vi "Teleop.vi"(10 "Match Info":T1={"Autonomous Elapsed Seconds"=0.0, "TeleOp Elapsed Seconds"=0.0, "Disabled Elapsed Seconds"=0.0, "Visited Autonomous"=FALSE, "Visited TeleOp"=FALSE, "Visited Disabled"=FALSE, "Autonomous Settings"={"Autonomous Style"=enum."Independent", "VI Refnum"=refnum}}, 11 "Call Context":T2) -> ()   [LabVIEW 2016]
doc: "This VI is called for each TeleOp packet received from the DS where the robot is not disabled. It is often used to read from the joysticks and update I/O or to update setpoints for timed control loops. It should complete and return within 20 milliseconds or it may miss DS packets."
uses:
  <vilib>/Rock Robotics/WPI/DriverStation/WPI_DriverStationDerivedRobotMode.ctl
  <vilib>/Rock Robotics/WPI/DriverStation/WPI_DriverStationMatch Info.ctl
  <vilib>/Rock Robotics/WPI/Utilities/WPI_GetSetVariantRefNum.vi
  <vilib>/Rock Robotics/Network Tables/NT Write Numeric Array.vi
  <vilib>/Rock Robotics/Network Tables/NT Read Boolean.vi
  <vilib>/Rock Robotics/Network Tables/NT Write Number.vi
  <vilib>/Rock Robotics/Network Tables/NT Write Boolean.vi
  <vilib>/Rock Robotics/Network Tables/NT Read Number.vi
  <vilib>/Rock Robotics/Network Tables/NT Write Boolean Array.vi
panel:
  out "Limit?":bool
  out "Lift Bottom":dbl
  out "Lift Top":dbl
  out "Sample Boolean 1":bool
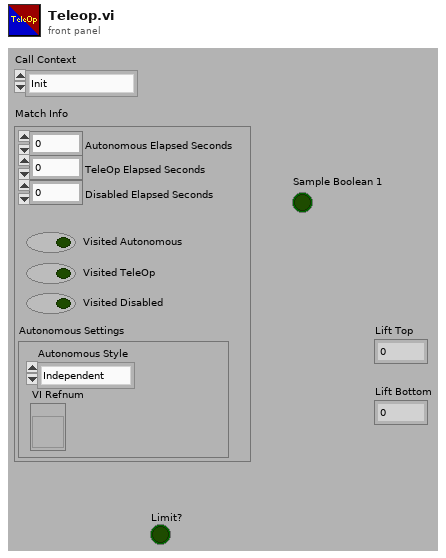
[diagram p1: front panel]
types:
  T1 = typedef "WPI_DriverStationMatch Info.ctl" = cluster{"Autonomous Elapsed Seconds":dbl, "TeleOp Elapsed Seconds":dbl, "Disabled Elapsed Seconds":dbl, "Visited Autonomous":bool, "Visited TeleOp":bool, "Visited Disabled":bool, "Autonomous Settings":cluster{"Autonomous Style":enum16{"Iterative", "Independent"}, "VI Refnum":refnum<vi>}}
  T2 = typedef "WPI_DriverStationDerivedRobotMode.ctl" = enum16{"Init", "Execute", "Stop"}
  T3 = typedef "WPI_GyroDevRef.ctl" = cluster{"DevStatus":errorcluster, "Analog Channel":T4, "Offset":dbl, "Gain (VoltsPerDegree/Second)":dbl, "Gyro Type":enum16{"Analog", "XRS450"}, "Handle":i32, "SPI Bus":T5, "Device Found":bool, "Sample Rate":dbl, "Calibrate On Open":bool}
  T4 = typedef "FPGA_AIChannel.ctl" = enum8{"AI 0", "AI 1", "AI 2", "AI 3", "AI MXP 0", "AI MXP 1", "AI MXP 2", "AI MXP 3", "Invalid"}
  T5 = typedef "spi_bus.ctl" = enum16{"SPI On-Board, CS0", "SPI On-Board, CS1", "SPI On-Board, CS2", "SPI On-Board, CS3", "SPI MXP", "Invalid"}
  T6 = typedef "WPI_JoystickDevRef.ctl" = cluster{"Device":T7}
  T7 = typedef "WPI_JoystickDeviceEnum.ctl" = enum16{"USB 0", "USB 1", "USB 2", "USB 3", "USB 4", "USB 5"}
  T8 = cluster{"Buttons[0]":bool, "Buttons[1]":bool, "Buttons[2]":bool, "Buttons[3]":bool, "Buttons[4]":bool, "Buttons[5]":bool, "Buttons[6]":bool, "Buttons[7]":bool, "Buttons[8]":bool}
  T9 = typedef "WPI_DigitalInputDevRef.ctl" = cluster{"DevStatus":errorcluster, "DIO Channel":T10}
  T10 = typedef "FPGA_DIOChannel.ctl" = enum8{"DIO 0", "DIO 1", "DIO 2", "DIO 3", "DIO 4", "DIO 5", "DIO 6", "DIO 7", "DIO 8", "DIO 9", "DIO MXP 0", "DIO MXP 1", "DIO MXP 2", "DIO MXP 3", "DIO MXP 4", "DIO MXP 5", "DIO MXP 6", "DIO MXP 7", "DIO MXP 8", "DIO MXP 9", "DIO MXP 10", "DIO MXP 11", "DIO MXP 12", "DIO MXP 13", "DIO MXP 14", "DIO MXP 15", "SPI Port CS1", "SPI Port CS2", "SPI Port CS3", "SPI Port MISO", "SPI Port MOSI", "Invalid"}
  T11 = typedef "WPI_RobotDriveDevRef.ctl" = cluster{"DevStatus":errorcluster, "Motors[]":T12[], "Square Inputs":bool, "Max Output":dbl}
  T12 = typedef "WPI_MotorControlDeviceRef.ctl" = cluster{"DeviceStatus":errorcluster, "Type":T13, "PWM":cluster{"PWM Channel":T14, "DeadBand":T15}, "CAN":cluster{"Device Number":u8, "SetOutput VI Ref":variant, "GetOutput VI Ref":variant, "Enable VI Ref":variant, "Disable VI Ref":variant, "Data":variant}, "Invert":bool}
  T13 = typedef "WPI_MotorControlType.ctl" = enum16{"PWM", "CAN"}
  T14 = typedef "FPGA_DIOPWMChannel.ctl" = enum8{"PWM 0", "PWM 1", "PWM 2", "PWM 3", "PWM 4", "PWM 5", "PWM 6", "PWM 7", "PWM 8", "PWM 9", "PWM MXP 0", "PWM MXP 1", "PWM MXP 2", "PWM MXP 3", "PWM MXP 4", "PWM MXP 5", "PWM MXP 6", "PWM MXP 7", "PWM MXP 8", "PWM MXP 9", "Invalid"}
  T15 = typedef "WPI_PWMDeadband.ctl" = cluster{"Name":string, "maxPositivePwm":i32, "minPositivePwm":i32, "centerPwm":i32, "maxNegativePwm":i32, "minNegativePwm":i32, "angularRange":u16}
  T16 = cluster{"Axes[0]":dbl, "Axes[1]":dbl, "Axes[2]":dbl, "Axes[3]":dbl, "Axes[4]":dbl, "Axes[5]":dbl, "Axes[6]":dbl, "Axes[7]":dbl, "Axes[8]":dbl}
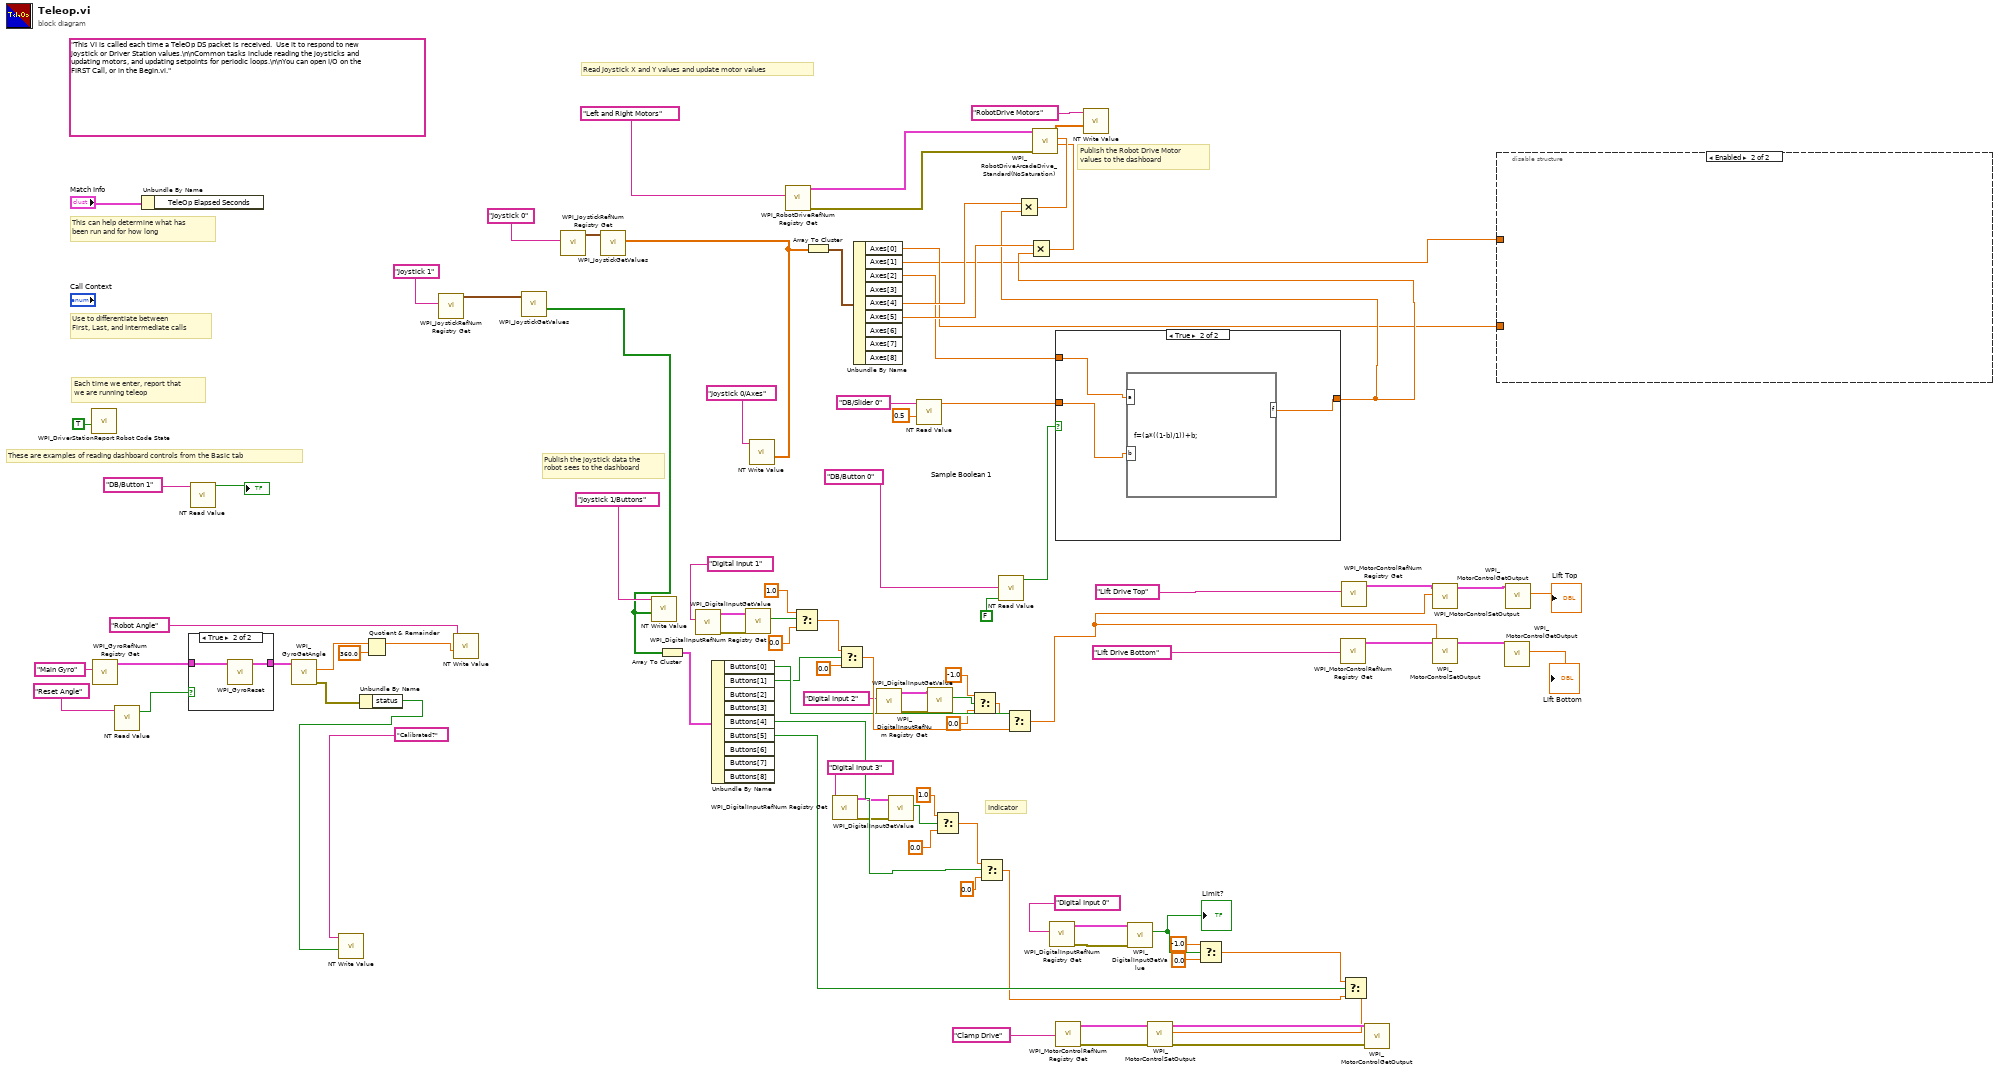
[diagram p0: block diagram]
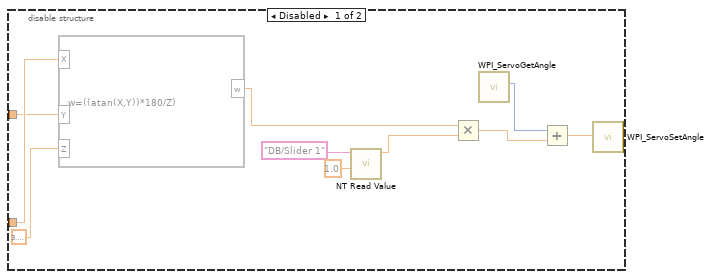
[diagram p2: hidden frame]
diagram:
  (unwired) "This VI is called each time a TeleOp DS packet is received.  Use it to respond to new joystick or Driver Station values.\n\nCommon tasks include reading the joysticks and updating motors, and updating setpoints for periodic loops.\n\nYou can open I/O on the FIRST Call, or in the Begin.vi."
  # "Indicator"
  # "These are examples of reading dashboard controls from the Basic tab"
  # "Publish the Robot Drive Motor\nvalues to the dashboard"
  # "Publish the joystick data the\nrobot sees to the dashboard"
  # "Each time we enter, report that\nwe are running teleop"
  # "Use to differentiate between\nFirst, Last, and Intermediate calls"
  # "This can help determine what has\nbeen run and for how long"
  # "Read Joystick X and Y values and update motor values"
  n1 = call <vilib>:"WPI_DriverStationReport Robot Code State.vi"("TeleOp"=TRUE ("Autonomous")) -> ()  [unwired: 10 in, 1 out]
  n2 = call <vilib>:"WPI_GyroRefNum Registry Get.vi"("refnum name"="Main Gyro") -> ("GyroDevRef"=w61:T3)  [unwired: 9 in, 1 out]
  n3 = call-poly <vilib>:"NT Read Value.vi"("Name"="Reset Angle") -> ("Boolean"=w58:bool)  [unwired: 9 in, 1 out]
  n4 = Unbundle By Name("Match Info") -> ()  [unwired: 1 out]
  n5 = case shown="True" w58 {
    tunnel: [w97 w99] -> w65
    tunnel: w61 -> [w97 w98]
    frame False {
    }
    frame True {
      n6 = call <vilib>:"WPI_GyroReset.vi"("GyroDevRef"=w98) -> ("GyroDevRef"=w99:T3)  [unwired: 9 in, 1 out]
    }
  }
  n7 = call-poly <vilib>:"NT Read Value.vi"("Name"="DB/Button 1" ("refnum name")) -> ("Boolean"=→"Sample Boolean 1":bool)  [unwired: 9 in, 1 out]
  n8 = call <vilib>:"WPI_GyroGetAngle.vi"("GyroDevRef"=w65) -> ("error out"=w63:errorcluster, "Angle"=w64:dbl)  [unwired: 7 in, 2 out]
  n9 = Unbundle By Name(w63) -> ("status"=w44:bool)
  n10 = call-poly <vilib>:"NT Write Value.vi"("Boolean"=w44, "Name"="Calibrated?") -> ()  [unwired: 9 in, 1 out]
  n11 = Quotient & Remainder(x=w64, y=360.0) -> (x-y*floor(x/y)=w60:dbl)  [unwired: 1 out]
  n12 = call <vilib>:"WPI_JoystickRefNum Registry Get.vi"("refnum name"="Joystick 1") -> ("JoystickDevRef"=w36:T6)  [unwired: 9 in, 1 out]
  n13 = call-poly <vilib>:"NT Write Value.vi"("Numeric"=w60, "Name"="Robot Angle") -> ()  [unwired: 9 in, 1 out]
  n14 = call <vilib>:"WPI_JoystickGetValues.vi"("JoystickDevRef"=w36) -> ("Buttons"=w35:bool[])  [unwired: 6 in, 4 out]
  n15 = call <vilib>:"WPI_JoystickRefNum Registry Get.vi"("refnum name"="Joystick 0") -> ("JoystickDevRef"=w93:T6)  [unwired: 1 in, 9 out]
  n16 = call <vilib>:"WPI_JoystickGetValues.vi"("JoystickDevRef"=w93) -> ("Axes"=w54:dbl[])  [unwired: 6 in, 4 out]
  n17 = call-poly <vilib>:"NT Write Value.vi"("Boolean Array"=w35, "Name"="Joystick 1/Buttons") -> ()  [unwired: 9 in, 1 out]
  n18 = Array To Cluster(array=w35) -> (cluster=w55:T8)
  n19 = call <vilib>:"WPI_DigitalInputRefNum Registry Get.vi"("refnum name"="Digital Input 1") -> ("error out"=w17:errorcluster, "DigitalInputDevRef"=w18:T9)  [unwired: 9 in]
  n20 = Unbundle By Name(w55) -> ("Buttons[0]"=w38:bool, "Buttons[1]"=w14:bool, "Buttons[4]"=w11:bool, "Buttons[5]"=w13:bool)  [unwired: 5 out]
  n21 = call <vilib>:"WPI_DigitalInputGetValue.vi"("error in (no error)"=w17, "DigitalInputDevRef"=w18) -> ("Value"=w16:bool)  [unwired: 7 in, 2 out]
  n22 = call-poly <vilib>:"NT Write Value.vi"("Numeric Array"=w54, "Name"="Joystick 0/Axes") -> ()  [unwired: 9 in, 1 out]
  n23 = call <vilib>:"WPI_RobotDriveRefNum Registry Get.vi"("refnum name"="Left and Right Motors") -> ("error out"=w50:errorcluster, "RobotDriveDevRef"=w94:T11)  [unwired: 1 in, 8 out]
  n24 = Select(t=1.0, s=w16, f=0.0) -> (s? t:f=w27:dbl)
  n25 = Array To Cluster(array=w54) -> (cluster=w53:T16)
  n26 = call <vilib>:"WPI_DigitalInputRefNum Registry Get.vi"("refnum name"="Digital Input 3") -> ("error out"=w1:errorcluster, "DigitalInputDevRef"=w10:T9)  [unwired: 9 in]
  n27 = Select(t=w27, s=w14, f=0.0) -> (s? t:f=w72:dbl)
  n28 = Unbundle By Name(w53) -> ("Axes[0]"=w40:dbl, "Axes[1]"=w39:dbl, "Axes[2]"=w41:dbl, "Axes[4]"=w52:dbl, "Axes[5]"=w51:dbl)  [unwired: 4 out]
  n29 = call <vilib>:"WPI_DigitalInputRefNum Registry Get.vi"("refnum name"="Digital Input 2") -> ("error out"=w21:errorcluster, "DigitalInputDevRef"=w22:T9)  [unwired: 9 in]
  n30 = call <vilib>:"WPI_DigitalInputGetValue.vi"("error in (no error)"=w1, "DigitalInputDevRef"=w10) -> ("Value"=w8:bool)  [unwired: 7 in, 2 out]
  n31 = call-poly <vilib>:"NT Read Value.vi"("Default Value"=0.5, "Name"="DB/Slider 0" ("refnum name")) -> ("Numeric"=w46:dbl)  [unwired: 8 in, 1 out]
  n32 = call <vilib>:"WPI_DigitalInputGetValue.vi"("error in (no error)"=w21, "DigitalInputDevRef"=w22) -> ("Value"=w20:bool)  [unwired: 7 in, 2 out]
  n33 = Select(t=1.0, s=w8, f=0.0) -> (s? t:f=w5:dbl)
  n34 = Select(t=-1.0, s=w20, f=0.0) -> (s? t:f=w28:dbl)
  n35 = Select(t=w5, s=w11, f=0.0) -> (s? t:f=w2:dbl)
  n36 = call-poly <vilib>:"NT Read Value.vi"("Default Value"=FALSE, "Name"="DB/Button 0" ("refnum name")) -> ("Boolean"=w48:bool)  [unwired: 8 in, 1 out]
  n37 = Select(t=w28, s=w38, f=w72) -> (s? t:f=w73:dbl)
  n38 = call <vilib>:"WPI_DigitalInputRefNum Registry Get.vi"("refnum name"="Digital Input 0") -> ("error out"=w32:errorcluster, "DigitalInputDevRef"=w34:T9)  [unwired: 9 in]
  n39 = case shown="True" w48 {
    tunnel: [w100 w101] -> w43
    tunnel: w46 -> [w100 w102]
    tunnel: w41 -> [_ w103]
    frame False {
    }
    frame True {
      n40 = formula code="f=(a*((1-b)/1))+b;"("a"=w103, "b"=w102) -> ("f"=w101:dbl)
    }
  }
  n41 = Multiply(x=w52, y=w43) -> (x*y=w83:dbl)
  n42 = Multiply(x=w51, y=w43) -> (x*y=w82:dbl)
  n43 = call <vilib>:"WPI_RobotDriveArcadeDrive_Standard(NoSaturation).vi"("error in (no error)"=w50, "Y axis value"=w82, "X axis value"=w83, "RobotDriveDevRef"=w94) -> ("Motor Values"=w86:dbl[])  [unwired: 7 out]
  n44 = call <vilib>:"WPI_MotorControlRefNum Registry Get.vi"("refnum name"="Clamp Drive") -> ("error out"=w71:errorcluster, "MotorControlDevRef"=w69:T12)  [unwired: 9 in]
  n45 = call-poly <vilib>:"NT Write Value.vi"("Numeric Array"=w86, "Name"="RobotDrive Motors") -> ()  [unwired: 9 in, 1 out]
  n46 = call <vilib>:"WPI_DigitalInputGetValue.vi"("error in (no error)"=w32, "DigitalInputDevRef"=w34) -> ("Value"=w30:bool)  [unwired: 7 in, 2 out]
  "Limit?" <- w30
  n47 = Select(t=-1.0, s=w30, f=0.0) -> (s? t:f=w3:dbl)
  n48 = call <vilib>:"WPI_MotorControlRefNum Registry Get.vi"("refnum name"="Lift Drive Bottom") -> ("MotorControlDevRef"=w78:T12)  [unwired: 9 in, 1 out]
  n49 = call <vilib>:"WPI_MotorControlRefNum Registry Get.vi"("refnum name"="Lift Drive Top") -> ("MotorControlDevRef"=w79:T12)  [unwired: 9 in, 1 out]
  n50 = Select(t=w3, s=w13, f=w2) -> (s? t:f=w29:dbl)
  n51 = call <vilib>:"WPI_MotorControlSetOutput.vi"("error in (no error)"=w71, "Output"=w29, "MotorControlDevRef"=w69) -> ("error out"=w68:errorcluster, "MotorControlDevRef"=w70:T12)  [unwired: 6 in, 1 out]
  n52 = call <vilib>:"WPI_MotorControlGetOutput.vi"("error in (no error)"=w68, "MotorControlDevRef"=w70) -> ()  [unwired: 7 in, 3 out]
  n53 = call <vilib>:"WPI_MotorControlSetOutput.vi"("Output"=w73, "MotorControlDevRef"=w79) -> ("MotorControlDevRef"=w80:T12)  [unwired: 7 in, 2 out]
  n54 = call <vilib>:"WPI_MotorControlSetOutput.vi"("Output"=w73, "MotorControlDevRef"=w78) -> ("MotorControlDevRef"=w81:T12)  [unwired: 7 in, 2 out]
  n55 = disable-structure shown="Enabled" {
    disable-tunnel: w40 -> [w113 _]
    disable-tunnel: w39 -> [w112 _]
    frame Disabled {
      n56 = formula code="w=((atan(X,Y))*180/Z)"("X"=w113, "Y"=w112, "Z"=3.141592653589793) -> ("w"=w107:dbl)
      n57 = call-poly <vilib>:"NT Read Value.vi"("Default Value"=1.0, "Name"="DB/Slider 1" ("refnum name")) -> ("Numeric"=w104:dbl)  [unwired: 8 in, 1 out]
      n58 = Multiply(x=w107, y=w104) -> (x*y=w108:dbl)
      n59 = call <vilib>:"WPI_ServoGetAngle.vi"() -> ("Angle"=w109:u16)  [unwired: 8 in, 2 out]
      n60 = Add(x=w109, y=w108) -> (x+y=w110:dbl)
      n61 = call <vilib>:"WPI_ServoSetAngle.vi"("Angle"=w110) -> ()  [unwired: 9 in, 2 out]
    }
    frame Enabled {
    }
  }
  n62 = call <vilib>:"WPI_MotorControlGetOutput.vi"("MotorControlDevRef"=w81) -> ("Output"=→"Lift Bottom":dbl)  [unwired: 8 in, 2 out]
  n63 = call <vilib>:"WPI_MotorControlGetOutput.vi"("MotorControlDevRef"=w80) -> ("Output"=→"Lift Top":dbl)  [unwired: 8 in, 2 out]
